vi "nD Nonlinear System Single Solution (VI).vi"(7 "accuracy":dbl=1e-08 format="%0.2e", 8 "F(X)":T1, 9 "data":variant, 10 "Start":dbl[](array[numeric]) format="%0.2f", 11 "h":dbl=1e-08 format="%0.2e") -> (0 "error":i32, 1 "ticks":u32, 2 "f(Zeroes)":dbl[](array[numeric]) format="%0.2f", 3 "Zeroes":dbl[](array[numeric]) format="%0.2f")   [LabVIEW 2017, in "NI_Gmath.lvlib"]
doc: "Determines the solutions of nonlinear systems of equations in n dimensions beginning with a starting point in n dimensions. You must manually select the polymorphic instance to use."
uses:
  NI_Gmath.lvlib
  functionRefnum nD.ctl
  Unit Vector (DBL).vi
  Matrix To Array - RM.vi
  Create Special Real Matrix.vi
  NI_AALBase.lvlib
  NI_AALPro.lvlib
  NI_Matrix.lvlib
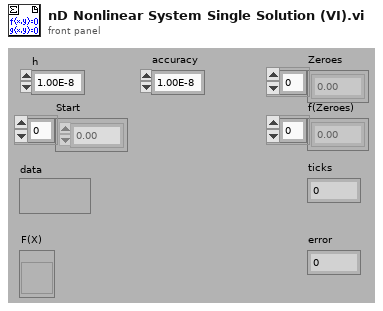
[diagram p1: front panel]
types:
  T1 = typedef "NI_Gmath.lvlib/functionRefnum nD.ctl" = refnum<vi>
  T2 = enum32{"Identity", "Diagonal", "Toepliz", "Vandermonde", "Companion"}
  T3 = typedef "NI_Matrix.lvlib/RealMatrix.ctl" = dbl[][]
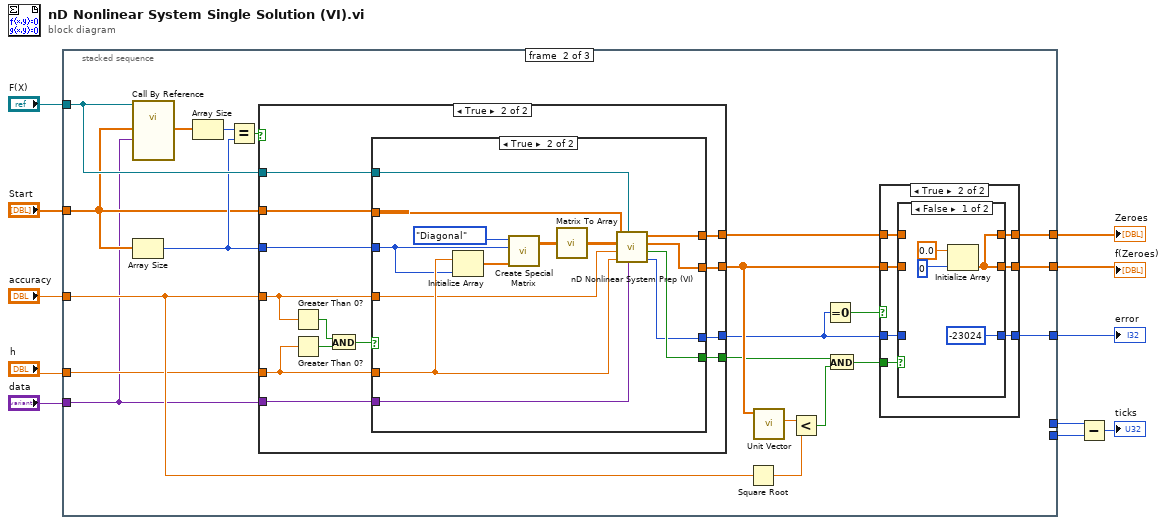
[diagram p0: block diagram]
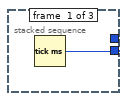
[diagram p2: hidden frame]
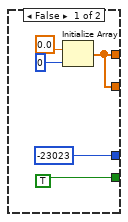
[diagram p3: hidden frame]
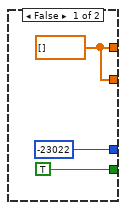
[diagram p4: hidden frame]
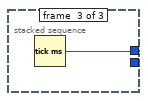
[diagram p7: hidden frame]
diagram:
  n1 = stacked-sequence {
    tunnel: [_ w33 _] -> w11
    tunnel: [_ w32 _] -> w10
    tunnel: [_ w28 _] -> w9
    tunnel: "accuracy" -> [_ w23 _]
    tunnel: "data" -> [_ w13 _]
    tunnel: "F(X)" -> [_ w17 _]
    tunnel: "Start" -> [_ w14 _]
    tunnel: "h" -> [_ w20 _]
    tunnel: [_ _ w86] -> w4
    tunnel: [w12 _ _] -> w3
    frame #0 {
      n2 = Tick Count (ms)() -> (millisecond timer value=w12:u32)
    }
    frame #1 {
      n3 = call-by-ref "?"(reference=w17, "variant"=w13, "X"=w14) -> ("F(X)"=w19:dbl[])  [unwired: 4 in, 2 out]
      n4 = Array Size(array=w14) -> (size(s)=w16:i32)
      n5 = Array Size(array=w19) -> (size(s)=w18:i32)
      n6 = Equal?(x=w18, y=w16) -> (x = y?=w15:bool)
      n7 = case shown="True" w15 {
        tunnel: [w36 w51] -> w31
        tunnel: [w36 w50] -> w29
        tunnel: [TRUE w49] -> w27
        tunnel: [-23023 w48] -> w25
        tunnel: w23 -> [_ w47]
        tunnel: w13 -> [_ w46]
        tunnel: w17 -> [_ w42]
        tunnel: w14 -> [_ w41]
        tunnel: w16 -> [_ w40]
        tunnel: w20 -> [_ w39]
        frame False {
          n8 = Initialize Array(0.0, 0) -> (w36:dbl[])
        }
        frame True {
          n9 = Greater Than 0?(x=w47) -> (x > 0?=w45:bool)
          n10 = Greater Than 0?(x=w39) -> (x > 0?=w44:bool)
          n11 = And(x=w45, y=w44) -> (x .and. y?=w43:bool)
          n12 = case shown="True" w43 {
            tunnel: w47 -> [_ w57]
            tunnel: w39 -> [_ w61]
            tunnel: [w52 w68] -> w50
            tunnel: [w52 w67] -> w51
            tunnel: [-23022 w55] -> w48
            tunnel: w41 -> [_ w66]
            tunnel: w40 -> [_ w60]
            tunnel: [TRUE w56] -> w49
            tunnel: w42 -> [_ w65]
            tunnel: w46 -> [_ w64]
            frame False {
              w52 = dbl[] [] ("initialized array")
            }
            frame True {
              n13 = Initialize Array(w61, w60) -> (w62:dbl[])
              n14 = call-poly "Create Special Matrix.vi"("matrix type"=T2."Diagonal", "matrix size"=w60, "Input Vector1"=w62) -> ("Special Matrix"=w59:T3)  [unwired: 1 in, 2 out]
              n15 = call-poly "Matrix To Array.vi"("Real Matrix"=w59) -> ("Real 2D Array"=w58:dbl[][])
              n16 = call "nD Nonlinear System Prep (VI).vi"("data"=w64, "F(X)"=w65, "h"=w61, "accuracy"=w57, "Diagonal h"=w58, "Start"=w66) -> (0:"error"=w55:i32, 1:"error"=w56:bool, "F(X)"=w67:dbl[], "Start New"=w68:dbl[])  [unwired: 1 in, 1 out]
            }
          }
        }
      }
      n17 = Square Root(x=w23) -> (sqrt(x)=w22:dbl)
      n18 = call-poly "Unit Vector.vi"("Input Vector"=w31) -> ("norm"=w21:dbl)  [unwired: 2 in, 8 out]
      n19 = Less?(x=w21, y=w22) -> (x < y?=w30:bool)
      n20 = Equal To 0?(x=w25) -> (x = 0?=w24:bool)
      n21 = And(x=w27, y=w30) -> (x .and. y?=w26:bool)
      n22 = case shown="True" w24 {
        tunnel: [w71 w78] -> w28
        tunnel: w29 -> [w71 w77]
        tunnel: w26 -> [_ w76]
        tunnel: w31 -> [w70 w75]
        tunnel: [w69 w74] -> w32
        tunnel: w25 -> [w69 w73]
        tunnel: [w70 w72] -> w33
        frame False {
        }
        frame True {
          n23 = case shown="False" w76 {
            tunnel: w77 -> [_ w85]
            tunnel: [w80 w85] -> w78
            tunnel: w75 -> [_ w84]
            tunnel: [w80 w84] -> w72
            tunnel: w73 -> [_ w83]
            tunnel: [-23024 w83] -> w74
            frame False {
              n24 = Initialize Array(0.0, 0) -> (w80:dbl[])
            }
            frame True {
            }
          }
        }
      }
    }
    frame #2 {
      n25 = Tick Count (ms)() -> (millisecond timer value=w86:u32)
    }
  }
  "Zeroes" <- w9
  "f(Zeroes)" <- w11
  "error" <- w10
  n26 = Subtract(x=w4, y=w3) -> (x-y=→"ticks":u32)
